vi "Serial Convert.vi"(8 "Range (V)":sgl=20.0 format="%#_13g", 11 "Raw serial buffer":string="\u0000\u0000\u0000\u0000\u0000\u0000\u0000\u0000\u0000\u0000\u0000\u0000\u0000\u0000\u0000\u0000\u0000\u0000") -> (0 "V6 (V)":sgl, 1 "V5 (V)":sgl, 2 "V4 (V)":sgl, 3 "V3 (V)":sgl, 4 "V7 (V)":sgl, 5 "V2 (V)":sgl, 6 "V8 (V)":sgl, 7 "V1 (V)":sgl)   [LabVIEW 2014]
panel:
  # "PN 19/12/2014"
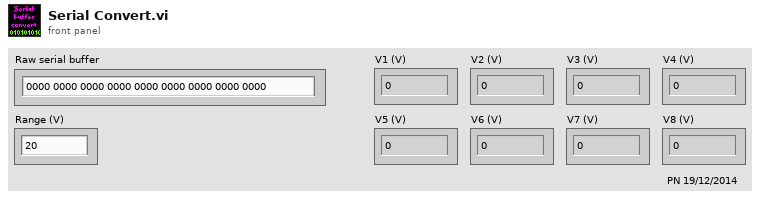
[diagram p1: front panel]
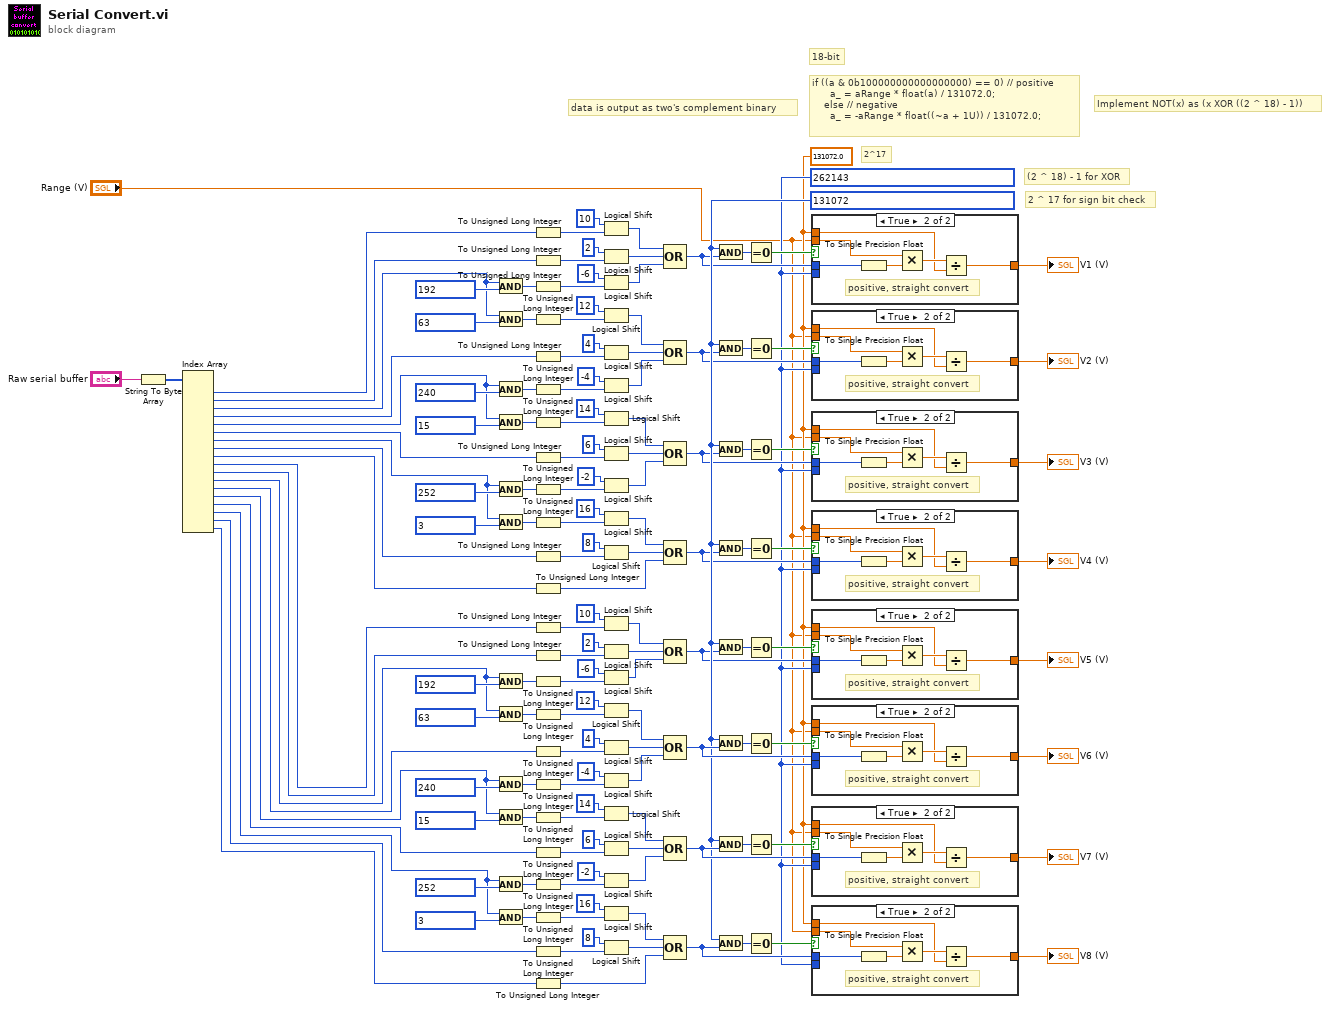
[diagram p0: block diagram]
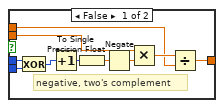
[diagram p2: hidden frame]
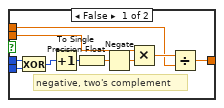
[diagram p3: hidden frame]
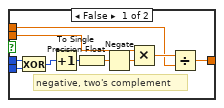
[diagram p4: hidden frame]
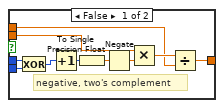
[diagram p5: hidden frame]
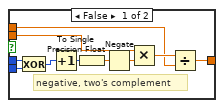
[diagram p6: hidden frame]
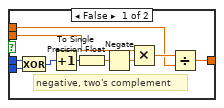
[diagram p7: hidden frame]
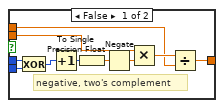
[diagram p8: hidden frame]
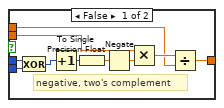
[diagram p9: hidden frame]
diagram:
  w21 = u32 262143
  w20 = sgl 131072.0
  w49 = u32 131072
  # "2 ^ 17 for sign bit check"
  # "(2 ^ 18) - 1 for XOR"
  # "Implement NOT(x) as (x XOR ((2 ^ 18) - 1))"
  # "18-bit"
  # "2^17"
  # "data is output as two's complement binary"
  # "if ((a & 0b100000000000000000) == 0) // positive\n      a_ = aRange * float(a) / 131072.0; \n    else // negative\n      a_ = -aRange * float((~a + 1U)) / 131072.0;"
  n1 = String To Byte Array(string="Raw serial buffer") -> (unsigned byte array=w143:u8[])
  n2 = Index Array(array=w143) -> (element #1=w147:u8, element #2=w144:u8, element #3=w135:u8, element #4=w131:u8, element #5=w123:u8, element #6=w118:u8, element #7=w111:u8, element #8=w106:u8, element #9=w102:u8, element #10=w48:u8, element #11=w47:u8, element #12=w46:u8, element #13=w45:u8, element #14=w44:u8, element #15=w43:u8, element #16=w42:u8, element #17=w41:u8, element #18=w40:u8)  [unwired: 18 in]
  n3 = And(x=w135, y=u8 192) -> (x .and. y?=w139:u8)
  n4 = And(x=w135, y=u8 63) -> (x .and. y?=w134:u8)
  n5 = And(x=w123, y=u8 240) -> (x .and. y?=w127:u8)
  n6 = And(x=w123, y=u8 15) -> (x .and. y?=w122:u8)
  n7 = And(x=w111, y=u8 252) -> (x .and. y?=w113:u8)
  n8 = And(x=w111, y=u8 3) -> (x .and. y?=w110:u8)
  n9 = And(x=w46, y=u8 192) -> (x .and. y?=w55:u8)
  n10 = And(x=w46, y=u8 63) -> (x .and. y?=w59:u8)
  n11 = And(x=w44, y=u8 240) -> (x .and. y?=w65:u8)
  n12 = And(x=w44, y=u8 15) -> (x .and. y?=w69:u8)
  n13 = And(x=w42, y=u8 252) -> (x .and. y?=w77:u8)
  n14 = And(x=w42, y=u8 3) -> (x .and. y?=w79:u8)
  n15 = To Unsigned Long Integer(number=w147) -> (unsigned 32bit integer=w142:u32)
  n16 = To Unsigned Long Integer(number=w144) -> (unsigned 32bit integer=w141:u32)
  n17 = To Unsigned Long Integer(number=w139) -> (unsigned 32bit integer=w17:u32)
  n18 = To Unsigned Long Integer(number=w134) -> (unsigned 32bit integer=w133:u32)
  n19 = To Unsigned Long Integer(number=w131) -> (unsigned 32bit integer=w130:u32)
  n20 = To Unsigned Long Integer(number=w127) -> (unsigned 32bit integer=w11:u32)
  n21 = To Unsigned Long Integer(number=w122) -> (unsigned 32bit integer=w120:u32)
  n22 = To Unsigned Long Integer(number=w118) -> (unsigned 32bit integer=w116:u32)
  n23 = To Unsigned Long Integer(number=w113) -> (unsigned 32bit integer=w7:u32)
  n24 = To Unsigned Long Integer(number=w110) -> (unsigned 32bit integer=w108:u32)
  n25 = To Unsigned Long Integer(number=w106) -> (unsigned 32bit integer=w104:u32)
  n26 = To Unsigned Long Integer(number=w102) -> (unsigned 32bit integer=w101:u32)
  n27 = To Unsigned Long Integer(number=w48) -> (unsigned 32bit integer=w52:u32)
  n28 = To Unsigned Long Integer(number=w47) -> (unsigned 32bit integer=w53:u32)
  n29 = To Unsigned Long Integer(number=w55) -> (unsigned 32bit integer=w13:u32)
  n30 = To Unsigned Long Integer(number=w59) -> (unsigned 32bit integer=w60:u32)
  n31 = To Unsigned Long Integer(number=w45) -> (unsigned 32bit integer=w62:u32)
  n32 = To Unsigned Long Integer(number=w65) -> (unsigned 32bit integer=w5:u32)
  n33 = To Unsigned Long Integer(number=w69) -> (unsigned 32bit integer=w71:u32)
  n34 = To Unsigned Long Integer(number=w43) -> (unsigned 32bit integer=w74:u32)
  n35 = To Unsigned Long Integer(number=w77) -> (unsigned 32bit integer=w2:u32)
  n36 = To Unsigned Long Integer(number=w79) -> (unsigned 32bit integer=w81:u32)
  n37 = To Unsigned Long Integer(number=w41) -> (unsigned 32bit integer=w84:u32)
  n38 = To Unsigned Long Integer(number=w40) -> (unsigned 32bit integer=w86:u32)
  n39 = Logical Shift(y=i16 10, x=w142) -> (x << y=w137:u32)
  n40 = Logical Shift(y=i16 2, x=w141) -> (x << y=w138:u32)
  n41 = Logical Shift(y=i16 -6, x=w17) -> (x << y=w16:u32)
  n42 = Logical Shift(y=i16 12, x=w133) -> (x << y=w126:u32)
  n43 = Logical Shift(y=i16 4, x=w130) -> (x << y=w125:u32)
  n44 = Logical Shift(y=i16 -4, x=w11) -> (x << y=w10:u32)
  n45 = Logical Shift(y=i16 14, x=w120) -> (x << y=w119:u32)
  n46 = Logical Shift(y=i16 6, x=w116) -> (x << y=w115:u32)
  n47 = Logical Shift(y=i16 -2, x=w7) -> (x << y=w8:u32)
  n48 = Logical Shift(y=i16 16, x=w108) -> (x << y=w107:u32)
  n49 = Logical Shift(y=i16 8, x=w104) -> (x << y=w103:u32)
  n50 = Logical Shift(y=i16 10, x=w52) -> (x << y=w57:u32)
  n51 = Logical Shift(y=i16 2, x=w53) -> (x << y=w56:u32)
  n52 = Logical Shift(y=i16 -6, x=w13) -> (x << y=w14:u32)
  n53 = Logical Shift(y=i16 12, x=w60) -> (x << y=w66:u32)
  n54 = Logical Shift(y=i16 4, x=w62) -> (x << y=w67:u32)
  n55 = Logical Shift(y=i16 -4, x=w5) -> (x << y=w4:u32)
  n56 = Logical Shift(y=i16 14, x=w71) -> (x << y=w72:u32)
  n57 = Logical Shift(y=i16 6, x=w74) -> (x << y=w75:u32)
  n58 = Logical Shift(y=i16 -2, x=w2) -> (x << y=w1:u32)
  n59 = Logical Shift(y=i16 16, x=w81) -> (x << y=w82:u32)
  n60 = Logical Shift(y=i16 8, x=w84) -> (x << y=w85:u32)
  n61 = Compound Arithmetic op=OR(w137, w138, w16) -> (w34:u32)
  n62 = Compound Arithmetic op=OR(w126, w125, w10) -> (w23:u32)
  n63 = Compound Arithmetic op=OR(w119, w115, w8) -> (w26:u32)
  n64 = Compound Arithmetic op=OR(w107, w103, w101) -> (w25:u32)
  n65 = Compound Arithmetic op=OR(w57, w56, w14) -> (w22:u32)
  n66 = Compound Arithmetic op=OR(w66, w67, w4) -> (w95:u32)
  n67 = Compound Arithmetic op=OR(w72, w75, w1) -> (w96:u32)
  n68 = Compound Arithmetic op=OR(w82, w85, w86) -> (w39:u32)
  n69 = And(x=w49, y=w34) -> (x .and. y?=w100:u32)
  n70 = And(x=w49, y=w23) -> (x .and. y?=w99:u32)
  n71 = And(x=w49, y=w26) -> (x .and. y?=w98:u32)
  n72 = And(x=w49, y=w25) -> (x .and. y?=w97:u32)
  n73 = And(x=w49, y=w22) -> (x .and. y?=w87:u32)
  n74 = And(x=w49, y=w95) -> (x .and. y?=w88:u32)
  n75 = And(x=w49, y=w96) -> (x .and. y?=w89:u32)
  n76 = And(x=w49, y=w39) -> (x .and. y?=w94:u32)
  n77 = Equal To 0?(x=w100) -> (x = 0?=w35:bool)
  n78 = Equal To 0?(x=w99) -> (x = 0?=w24:bool)
  n79 = Equal To 0?(x=w98) -> (x = 0?=w33:bool)
  n80 = Equal To 0?(x=w97) -> (x = 0?=w28:bool)
  n81 = Equal To 0?(x=w87) -> (x = 0?=w27:bool)
  n82 = Equal To 0?(x=w88) -> (x = 0?=w90:bool)
  n83 = Equal To 0?(x=w89) -> (x = 0?=w91:bool)
  n84 = Equal To 0?(x=w94) -> (x = 0?=w38:bool)
  n85 = case shown="True" w35 {
    tunnel: "Range (V)" -> [w155 w162]
    tunnel: w20 -> [w154 w160]
    tunnel: w34 -> [w150 w164]
    tunnel: [w153 w159] -> w36
    tunnel: w21 -> [w149 _]
    frame False {
      # "negative, two's complement"
      n86 = Exclusive Or(1:w149, 2:w150) -> (0:w151:u32)
      n87 = Increment(x=w151) -> (x+1=w156:u32)
      n88 = To Single Precision Float(number=w156) -> (single precision float=w158:sgl)
      n89 = Negate(x=w158) -> (-x=w152:sgl)
      n90 = Multiply(x=w155, y=w152) -> (x*y=w157:sgl)
      n91 = Divide(x=w157, y=w154) -> (x/y=w153:sgl)
    }
    frame True {
      # "positive, straight convert"
      n92 = To Single Precision Float(number=w164) -> (single precision float=w163:sgl)
      n93 = Multiply(x=w162, y=w163) -> (x*y=w161:sgl)
      n94 = Divide(x=w161, y=w160) -> (x/y=w159:sgl)
    }
  }
  "V1 (V)" <- w36
  n95 = case shown="True" w24 {
    tunnel: "Range (V)" -> [w171 w178]
    tunnel: w20 -> [w170 w176]
    tunnel: w23 -> [w166 w180]
    tunnel: [w169 w175] -> w31
    tunnel: w21 -> [w165 _]
    frame False {
      # "negative, two's complement"
      n96 = Exclusive Or(1:w165, 2:w166) -> (0:w167:u32)
      n97 = Increment(x=w167) -> (x+1=w172:u32)
      n98 = To Single Precision Float(number=w172) -> (single precision float=w174:sgl)
      n99 = Negate(x=w174) -> (-x=w168:sgl)
      n100 = Multiply(x=w171, y=w168) -> (x*y=w173:sgl)
      n101 = Divide(x=w173, y=w170) -> (x/y=w169:sgl)
    }
    frame True {
      # "positive, straight convert"
      n102 = To Single Precision Float(number=w180) -> (single precision float=w179:sgl)
      n103 = Multiply(x=w178, y=w179) -> (x*y=w177:sgl)
      n104 = Divide(x=w177, y=w176) -> (x/y=w175:sgl)
    }
  }
  "V2 (V)" <- w31
  n105 = case shown="True" w33 {
    tunnel: "Range (V)" -> [w187 w194]
    tunnel: w20 -> [w186 w192]
    tunnel: w26 -> [w182 w196]
    tunnel: [w185 w191] -> w32
    tunnel: w21 -> [w181 _]
    frame False {
      # "negative, two's complement"
      n106 = Exclusive Or(1:w181, 2:w182) -> (0:w183:u32)
      n107 = Increment(x=w183) -> (x+1=w188:u32)
      n108 = To Single Precision Float(number=w188) -> (single precision float=w190:sgl)
      n109 = Negate(x=w190) -> (-x=w184:sgl)
      n110 = Multiply(x=w187, y=w184) -> (x*y=w189:sgl)
      n111 = Divide(x=w189, y=w186) -> (x/y=w185:sgl)
    }
    frame True {
      # "positive, straight convert"
      n112 = To Single Precision Float(number=w196) -> (single precision float=w195:sgl)
      n113 = Multiply(x=w194, y=w195) -> (x*y=w193:sgl)
      n114 = Divide(x=w193, y=w192) -> (x/y=w191:sgl)
    }
  }
  "V3 (V)" <- w32
  n115 = case shown="True" w28 {
    tunnel: "Range (V)" -> [w203 w210]
    tunnel: w20 -> [w202 w208]
    tunnel: w25 -> [w198 w212]
    tunnel: [w201 w207] -> w30
    tunnel: w21 -> [w197 _]
    frame False {
      # "negative, two's complement"
      n116 = Exclusive Or(1:w197, 2:w198) -> (0:w199:u32)
      n117 = Increment(x=w199) -> (x+1=w204:u32)
      n118 = To Single Precision Float(number=w204) -> (single precision float=w206:sgl)
      n119 = Negate(x=w206) -> (-x=w200:sgl)
      n120 = Multiply(x=w203, y=w200) -> (x*y=w205:sgl)
      n121 = Divide(x=w205, y=w202) -> (x/y=w201:sgl)
    }
    frame True {
      # "positive, straight convert"
      n122 = To Single Precision Float(number=w212) -> (single precision float=w211:sgl)
      n123 = Multiply(x=w210, y=w211) -> (x*y=w209:sgl)
      n124 = Divide(x=w209, y=w208) -> (x/y=w207:sgl)
    }
  }
  "V4 (V)" <- w30
  n125 = case shown="True" w27 {
    tunnel: "Range (V)" -> [w219 w226]
    tunnel: w20 -> [w218 w224]
    tunnel: w22 -> [w214 w228]
    tunnel: [w217 w223] -> w29
    tunnel: w21 -> [w213 _]
    frame False {
      # "negative, two's complement"
      n126 = Exclusive Or(1:w213, 2:w214) -> (0:w215:u32)
      n127 = Increment(x=w215) -> (x+1=w220:u32)
      n128 = To Single Precision Float(number=w220) -> (single precision float=w222:sgl)
      n129 = Negate(x=w222) -> (-x=w216:sgl)
      n130 = Multiply(x=w219, y=w216) -> (x*y=w221:sgl)
      n131 = Divide(x=w221, y=w218) -> (x/y=w217:sgl)
    }
    frame True {
      # "positive, straight convert"
      n132 = To Single Precision Float(number=w228) -> (single precision float=w227:sgl)
      n133 = Multiply(x=w226, y=w227) -> (x*y=w225:sgl)
      n134 = Divide(x=w225, y=w224) -> (x/y=w223:sgl)
    }
  }
  "V5 (V)" <- w29
  n135 = case shown="True" w90 {
    tunnel: "Range (V)" -> [w235 w242]
    tunnel: w20 -> [w234 w240]
    tunnel: w95 -> [w230 w244]
    tunnel: [w233 w239] -> w92
    tunnel: w21 -> [w229 _]
    frame False {
      # "negative, two's complement"
      n136 = Exclusive Or(1:w229, 2:w230) -> (0:w231:u32)
      n137 = Increment(x=w231) -> (x+1=w236:u32)
      n138 = To Single Precision Float(number=w236) -> (single precision float=w238:sgl)
      n139 = Negate(x=w238) -> (-x=w232:sgl)
      n140 = Multiply(x=w235, y=w232) -> (x*y=w237:sgl)
      n141 = Divide(x=w237, y=w234) -> (x/y=w233:sgl)
    }
    frame True {
      # "positive, straight convert"
      n142 = To Single Precision Float(number=w244) -> (single precision float=w243:sgl)
      n143 = Multiply(x=w242, y=w243) -> (x*y=w241:sgl)
      n144 = Divide(x=w241, y=w240) -> (x/y=w239:sgl)
    }
  }
  "V6 (V)" <- w92
  n145 = case shown="True" w91 {
    tunnel: "Range (V)" -> [w251 w258]
    tunnel: w20 -> [w250 w256]
    tunnel: w96 -> [w246 w260]
    tunnel: [w249 w255] -> w93
    tunnel: w21 -> [w245 _]
    frame False {
      # "negative, two's complement"
      n146 = Exclusive Or(1:w245, 2:w246) -> (0:w247:u32)
      n147 = Increment(x=w247) -> (x+1=w252:u32)
      n148 = To Single Precision Float(number=w252) -> (single precision float=w254:sgl)
      n149 = Negate(x=w254) -> (-x=w248:sgl)
      n150 = Multiply(x=w251, y=w248) -> (x*y=w253:sgl)
      n151 = Divide(x=w253, y=w250) -> (x/y=w249:sgl)
    }
    frame True {
      # "positive, straight convert"
      n152 = To Single Precision Float(number=w260) -> (single precision float=w259:sgl)
      n153 = Multiply(x=w258, y=w259) -> (x*y=w257:sgl)
      n154 = Divide(x=w257, y=w256) -> (x/y=w255:sgl)
    }
  }
  "V7 (V)" <- w93
  n155 = case shown="True" w38 {
    tunnel: "Range (V)" -> [w267 w274]
    tunnel: w20 -> [w266 w272]
    tunnel: w39 -> [w262 w276]
    tunnel: [w265 w271] -> w37
    tunnel: w21 -> [w261 _]
    frame False {
      # "negative, two's complement"
      n156 = Exclusive Or(1:w261, 2:w262) -> (0:w263:u32)
      n157 = Increment(x=w263) -> (x+1=w268:u32)
      n158 = To Single Precision Float(number=w268) -> (single precision float=w270:sgl)
      n159 = Negate(x=w270) -> (-x=w264:sgl)
      n160 = Multiply(x=w267, y=w264) -> (x*y=w269:sgl)
      n161 = Divide(x=w269, y=w266) -> (x/y=w265:sgl)
    }
    frame True {
      # "positive, straight convert"
      n162 = To Single Precision Float(number=w276) -> (single precision float=w275:sgl)
      n163 = Multiply(x=w274, y=w275) -> (x*y=w273:sgl)
      n164 = Divide(x=w273, y=w272) -> (x/y=w271:sgl)
    }
  }
  "V8 (V)" <- w37
